vi "F Dwf Digital I2c Clear.vi"(8 "error in (no error)":errorcluster, 10 "pfFree":i32, 11 "hdwf":i32) -> (0 "error out":errorcluster, 2 "pfFree out":i32, 3 "function return":i32)   [LabVIEW 2019, in "Olasdwf.lvlib"]
doc: "DWFAPI int FDwfDigitalI2cClear(HDWF hdwf, int *pfFree);"
uses:
  Olasdwf.lvlib
  Windows/System32/dwf.dll
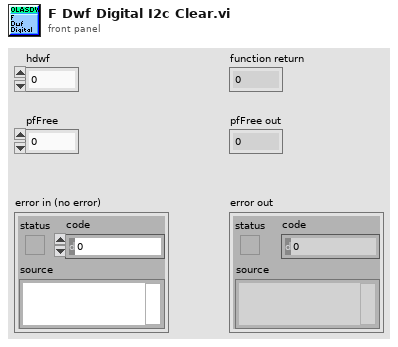
[diagram p1: front panel]
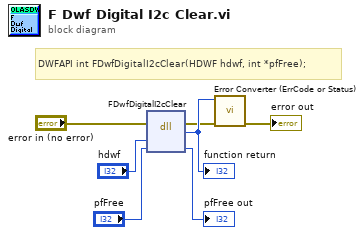
[diagram p0: block diagram]
diagram:
  # "DWFAPI int FDwfDigitalI2cClear(HDWF hdwf, int *pfFree);"
  n1 = dll-call lib="C:/Windows/System32/dwf.*" fn="FDwfDigitalI2cClear"(error in="error in (no error)", "hdwf"="hdwf", "pfFree"="pfFree") -> (error out=w2:errorcluster, w7:i32, "pfFree"=→"pfFree out":i32)  [unwired: 3 in, 1 out]
  "function return" <- w7
  n2 = call "Error Converter (ErrCode or Status).vi"("error in (no error)"=w2, "error code"=w7) -> ("error out"=→"error out":errorcluster)  [unwired: 9 in]
